vi "test Handle Is Valid Check.vi"(8 "error in (no error)":errorcluster, 11 "TestCase in":refnum<class "Memory Manager Tests.lvclass">) -> (0 "error out":errorcluster, 3 "TestCase out":refnum<class "Memory Manager Tests.lvclass">)   [LabVIEW 2024, in "Memory Manager Tests.lvclass"]
uses:
  Memory Manager Tests.lvclass
  <vilib>/Utility/file.llb/Application Directory.vi
  <vilib>/Utility/libraryn.llb/Check if File or Folder Exists.vi
  <vilib>/addons/_JKI Toolkits/VI Tester/TestCase.llb/TestCase.lvclass
  C:/Program Files/National Instruments/LabVIEW 2024/vi.lib/addons/_JKI Toolkits/VI Tester/TestCase.llb/TestCase.lvclass
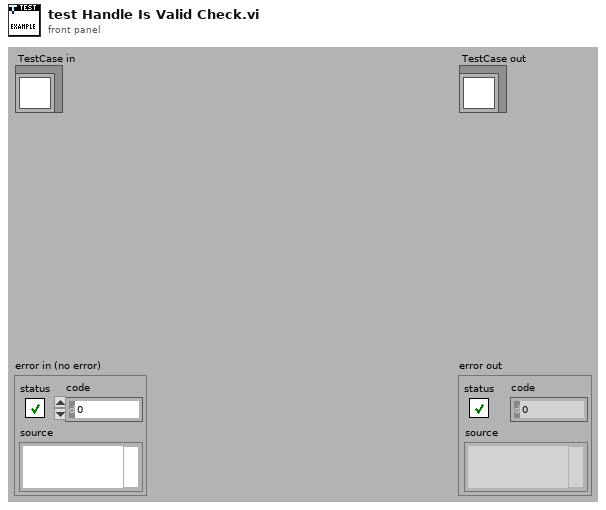
[diagram p1: front panel]
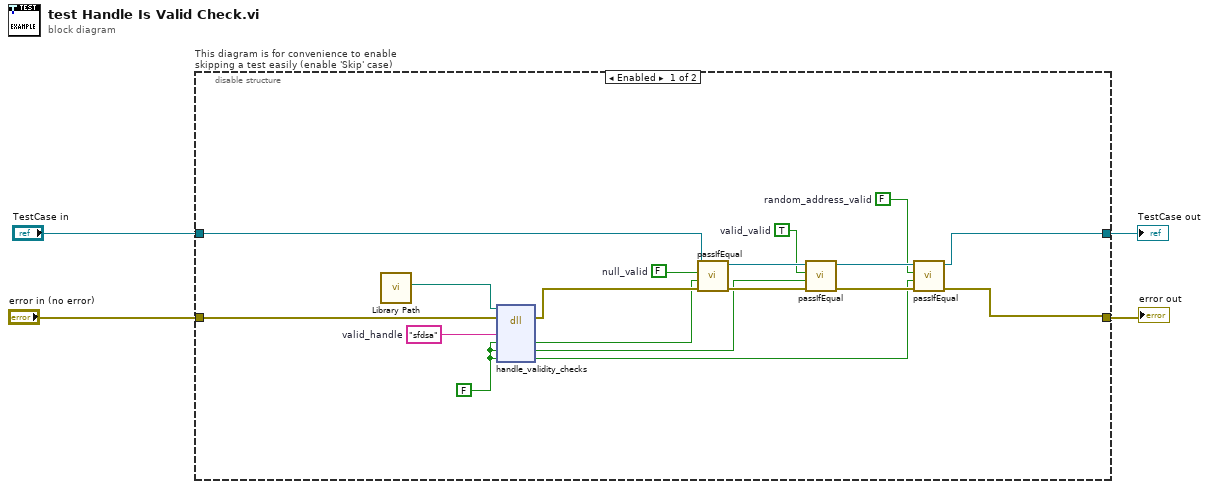
[diagram p0: block diagram]
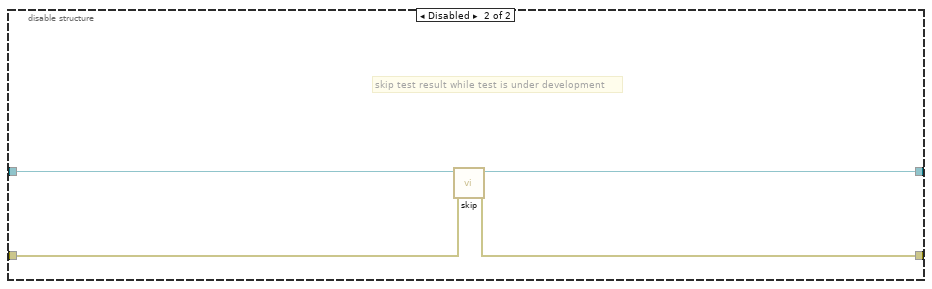
[diagram p2: hidden frame]
diagram:
  n1 = disable-structure "This diagram is for convenience to enable skipping a test easily (enable 'Skip' case)" shown="Enabled" {
    disable-tunnel: "TestCase in" -> [w22 w26]
    disable-tunnel: [w14 w24] -> w1
    disable-tunnel: [w15 w25] -> w3
    disable-tunnel: "error in (no error)" -> [w19 w23]
    frame Enabled {
      w5 = FALSE  # null_valid
      w6 = TRUE  # valid_valid
      w7 = FALSE  # random_address_valid
      w16 = "sfdsa"  # valid_handle
      w17 = FALSE
      n2 = call "Library Path.vi"() -> ("Library Path"=w20:path)  [unwired: 11 in]
      n3 = dll-call lib="C:/Users/JamesMcNally/Documents/RustInterop/Rust-LabVIEW-Interop/target/debug/labview_test_library.dll" fn="handle_validity_checks"(path in=w20, error in=w19, "valid_handle"=w16, "null_valid"=w17, "valid_valid"=w17, "random_address_valid"=w17) -> (error out=w18:errorcluster, "null_valid"=w10:bool, "valid_valid"=w9:bool, "random_address_valid"=w8:bool)  [unwired: 3 in, 1 out]
      n4 = call-dynamic "passIfEqual.vi"("error in (no error)"=w18, "y"=w10, "x"=w5, "TestCase in"=w22) -> ("error out"=w21:errorcluster, "TestCase out"=w12:refnum<class "Memory Manager Tests.lvclass">)  [unwired: 6 in]
      n5 = call-dynamic "passIfEqual.vi"("error in (no error)"=w21, "y"=w9, "x"=w6, "TestCase in"=w12) -> ("error out"=w13:errorcluster, "TestCase out"=w11:refnum<class "Memory Manager Tests.lvclass">)  [unwired: 6 in]
      n6 = call-dynamic "passIfEqual.vi"("error in (no error)"=w13, "y"=w8, "x"=w7, "TestCase in"=w11) -> ("error out"=w15:errorcluster, "TestCase out"=w14:refnum<class "Memory Manager Tests.lvclass">)  [unwired: 6 in]
    }
    frame Disabled {
      # "skip test result while test is under development"
      n7 = call <vilib>:"skip.vi"("error in (no error)"=w23, "TestCase in"=w26) -> ("error out"=w25:errorcluster, "TestCase out"=w24:refnum<class "Memory Manager Tests.lvclass">)  [unwired: 8 in]
    }
  }
  "error out" <- w3
  "TestCase out" <- w1
